vi "TEST_L0_COMPLETE_(ALL).vi"() -> ()   [LabVIEW 2012]
uses:
  <vilib>/Utility/NIReport.llb/NI_report.lvclass
  <vilib>/Utility/NIReport.llb/HTML/NI_HTML.lvclass
panel:
  in  "scripts executing filename":string="test.bat"
  in  "scripts directory":path=path "C:/Users/omartinez/Desktop"
  in  "Delay Test":bool=TRUE
  in  "Baseline":bool=TRUE
  in  "Majority Test":bool=TRUE
  in  "SumNAdder\n      Test":bool=TRUE
  in  "Sum Test":bool=TRUE
  in  "Instrument VISA in":T1={"AWG VISA"="AgilentGen1", "Oscilloscope  VISA "="AgilentOsc", "Integration Board IP"="172.16.17.47", "connection ID"=refnum, "report out"=refnum, "report file path"=path "C:/Users/omartinez/Desktop/L0nL1_Results"}
  out "Instrument VISA out":T1={"AWG VISA"="AgilentGen1", "Oscilloscope  VISA "="AgilentOsc", "Integration Board IP"="172.16.17.47", "connection ID"=refnum, "report out"=refnum, "report file path"=path "C:/Users/omartinez/Desktop/L0nL1_Results"}
  out "error out":errorcluster
  in  "error in":errorcluster
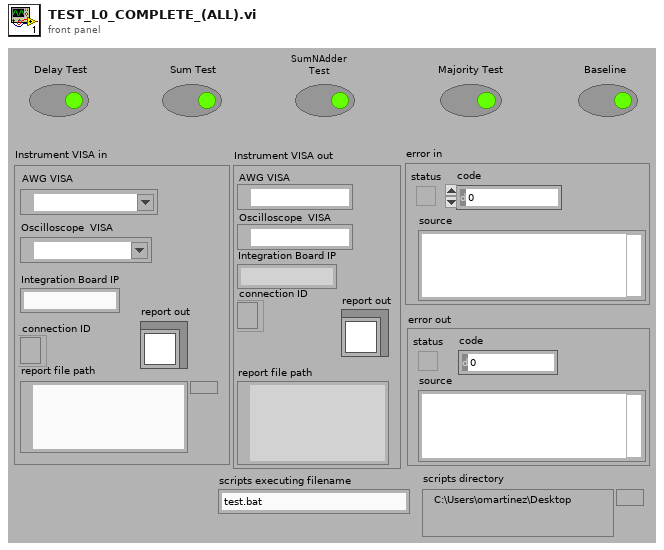
[diagram p1: front panel]
types:
  T1 = cluster{"AWG VISA":refnum<visa-resource-name>, "Oscilloscope  VISA ":refnum<visa-resource-name>, "Integration Board IP":string, "connection ID":refnum<k5>, "report out":refnum<class "NI_report.lvclass">, "report file path":path}
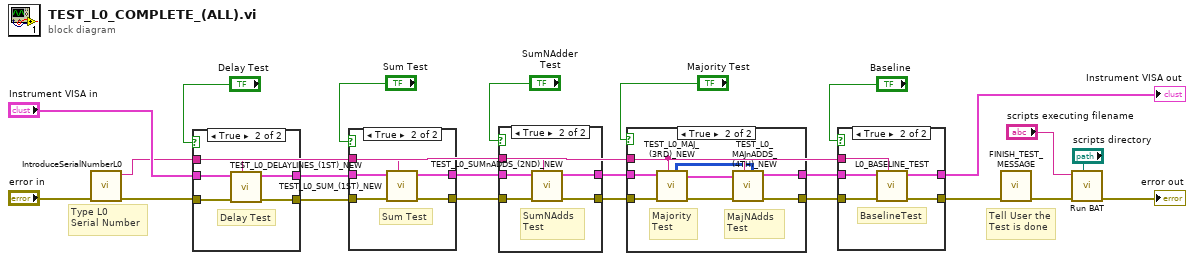
[diagram p0: block diagram]
diagram:
  # "Tell User the\nTest is done"
  # "Type L0\nSerial Number"
  n1 = call "IntroduceSerialNumberL0.vi"("error in"="error in") -> ("error out"=w8:errorcluster, "Serial Number"=w4:string)  [unwired: 9 in]
  n2 = case shown="True" "Delay Test" {
    tunnel: [w25 w30] -> w6
    tunnel: [w24 w29] -> w7
    tunnel: "Instrument VISA in" -> [w25 w28]
    tunnel: w8 -> [w24 w27]
    tunnel: w4 -> [_ w26]
    frame False {
    }
    frame True {
      # "Delay Test"
      n3 = call "TEST_L0_DELAYLINES_(1ST)_NEW.vi"("Serial Number"=w26, "error in (no error)"=w27, "Instrument VISA in"=w28) -> ("error out"=w29:errorcluster, "Instrument VISA out"=w30:T1)  [unwired: 7 in]
    }
  }
  n4 = case shown="True" "Sum Test" {
    tunnel: [w32 w37] -> w23
    tunnel: [w31 w36] -> w21
    tunnel: w6 -> [w32 w35]
    tunnel: w7 -> [w31 w34]
    tunnel: w4 -> [_ w33]
    frame False {
    }
    frame True {
      # "Sum Test"
      n5 = call "TEST_L0_SUM_(1ST)_NEW.vi"("Serial Number"=w33, "error in (no error)"=w34, "Instrument VISA in"=w35) -> ("error out"=w36:errorcluster, "Instrument VISA out"=w37:T1)  [unwired: 7 in]
    }
  }
  n6 = case shown="True" "SumNAdder\n      Test" {
    tunnel: w23 -> [w39 w41]
    tunnel: [w39 w42] -> w22
    tunnel: w21 -> [w38 w44]
    tunnel: [w38 w43] -> w20
    tunnel: w4 -> [_ w40]
    frame False {
    }
    frame True {
      # "SumNAdds\nTest"
      n7 = call "TEST_L0_SUMnADDS_(2ND)_NEW.vi"("Serial Number"=w40, "error in (no error)"=w44, "Instrument VISA in"=w41) -> ("error out"=w43:errorcluster, "Instrument VISA out"=w42:T1)  [unwired: 7 in]
    }
  }
  n8 = case shown="True" "Majority Test" {
    tunnel: w22 -> [w46 w54]
    tunnel: [w46 w52] -> w10
    tunnel: w20 -> [w45 w53]
    tunnel: [w45 w51] -> w11
    tunnel: w4 -> [_ w48]
    frame False {
    }
    frame True {
      # "MajNAdds\nTest"
      # "Majority\nTest"
      n9 = call "TEST_L0_MAJ_(3RD)_NEW.vi"("Serial Number"=w48, "error in"=w53, "Instrument VISA in"=w54) -> ("error out"=w49:errorcluster, "Instrument VISA out"=w50:T1, "ThresholdOut"=w47:i32[][])  [unwired: 6 in]
      n10 = call "TEST_L0_MAJnADDS_(4TH)_NEW.vi"("threshold"=w47, "Serial Number"=w48, "error in (no error)"=w49, "Instrument VISA in"=w50) -> ("error out"=w51:errorcluster, "Instrument VISA out"=w52:T1)  [unwired: 6 in]
    }
  }
  n11 = case shown="True" "Baseline" {
    tunnel: [w56 w58] -> w12
    tunnel: [w55 w61] -> w13
    tunnel: w10 -> [w56 w59]
    tunnel: w11 -> [w55 w60]
    tunnel: w4 -> [_ w57]
    frame False {
    }
    frame True {
      # "BaselineTest"
      n12 = call "L0_BASELINE_TEST.vi"("Serial Number"=w57, "error in"=w60, "Instrument VISA in"=w59) -> ("error out"=w61:errorcluster, "Instrument VISA out"=w58:T1)  [unwired: 7 in]
    }
  }
  "Instrument VISA out" <- w12
  n13 = call "FINISH_TEST_MESSAGE.vi"("error in"=w13) -> ("error out"=w15:errorcluster)  [unwired: 10 in]
  n14 = call "Run BAT.vi"("working directory"="scripts directory", "error in"=w15, "filename"="scripts executing filename") -> ("error out"=→"error out":errorcluster)  [unwired: 8 in]
